vi "main.vi"() -> ()   [LabVIEW 2015]
uses:
  <vilib>/addons/_office/_exclsub.llb/font.ctl
  Keithley 2000/Public/Configure/Configure AC Volts.vi
  <vilib>/Utility/NIReport.llb/NI_report.lvclass
  Agilent 3352X Series/Agilent 3352X Series.lvlib
  Keithley 2000/Keithley 2000.lvlib
  <vilib>/addons/_office/NI_ReportGenerationToolkit.lvlib
  <vilib>/Utility/NIReport.llb/Excel/NI_Excel.lvclass
panel:
  in  "连接":bool
  out "connecting":bool
  in  "原始记录":path=path "F:/电荷放大器/2692-原始记录.xls"
  in  "2010":refnum<visa-resource-name>="GPIB0::11::INSTR"
  in  "2000":refnum<visa-resource-name>="GPIB0::16::INSTR"
  in  "channel":i32=1 min=1 max=4 step=1
  in  "COM":i32=5
  in  "退出":bool
  in  "电平":enum16{"200mV~2V", "500mV~5V"}(ring)
  in  "33521A":refnum<visa-resource-name>="USB0::0x0957::0x1607::MY50003642::INSTR"
  in  "幅频特性":bool
  in  "增益档误差":bool
  in  "归一化误差":bool
  in  "线性误差":bool
  # "电 荷 放 大 器 自 动 化"
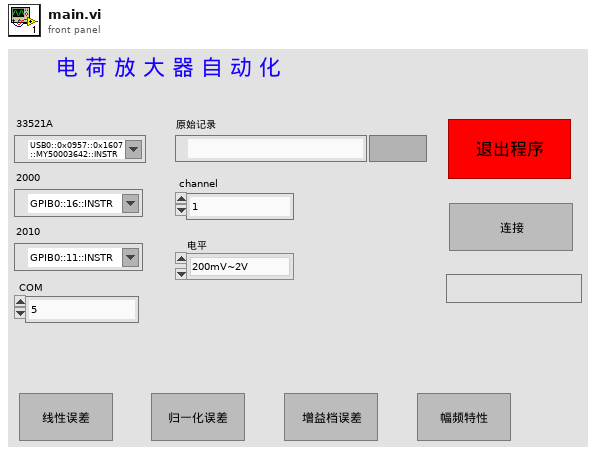
[diagram p1: front panel]
types:
  T1 = enum16{"maximized", "minimized", "normal", "no change"}
  T2 = enum16{"Standard Report", "HTML", "Word", "Excel"}
  T3 = cluster{"input float.":bool, "type":u16, "transd. mode":string, "transd. sens.":dbl, "unit":u16, "applied corr.":dbl, "position":string, "cable length":dbl, "supply":u16, "polarization":u16}
  T4 = typedef "NI_ReportGenerationToolkit.lvlib/font.ctl" = cluster{"font name":string, "font size":dbl, "bold":u16, "italic":u16, "underline":u16, "strike through":u16, "font color":u32}
  T5 = cluster{"high-pass (index)":u16, "low-pass (index)":u16, "outp. sens. (index)":u16, "output float.":bool}
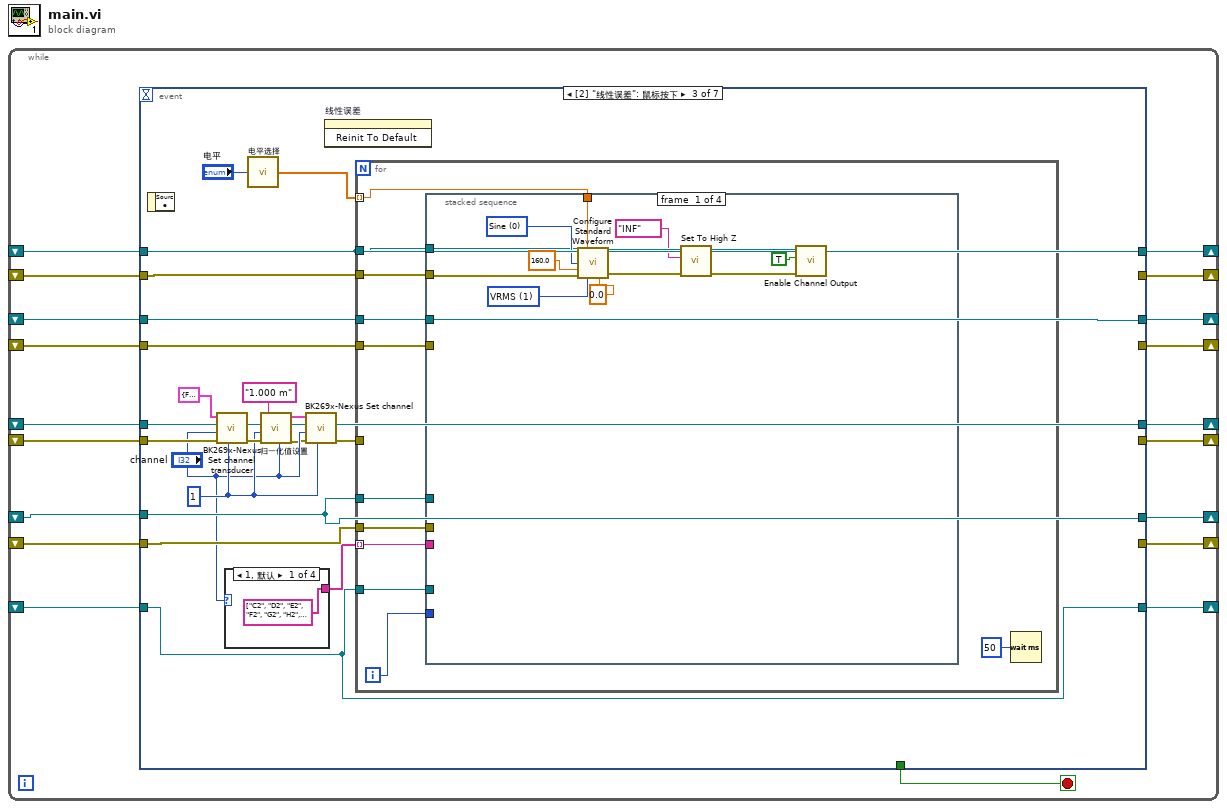
[diagram p0: block diagram]
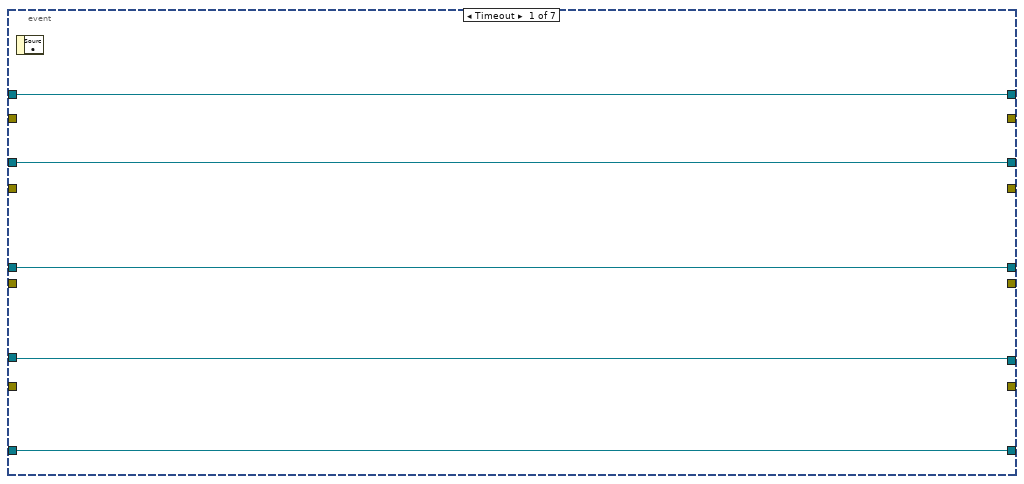
[diagram p2: hidden frame]
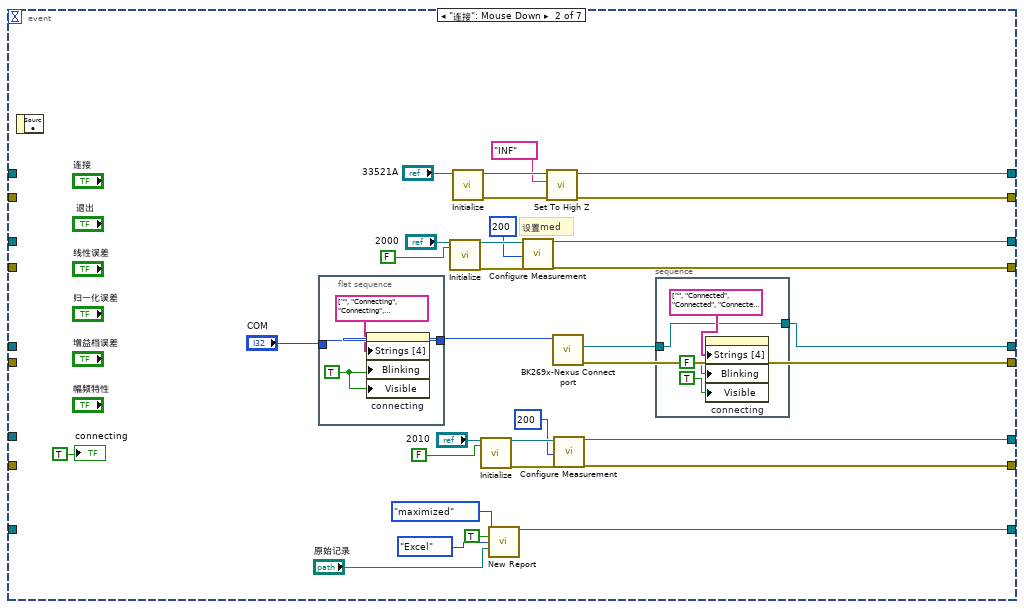
[diagram p3: hidden frame]
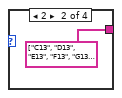
[diagram p4: hidden frame]
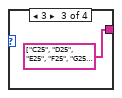
[diagram p5: hidden frame]
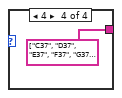
[diagram p6: hidden frame]
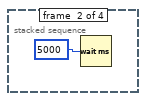
[diagram p7: hidden frame]
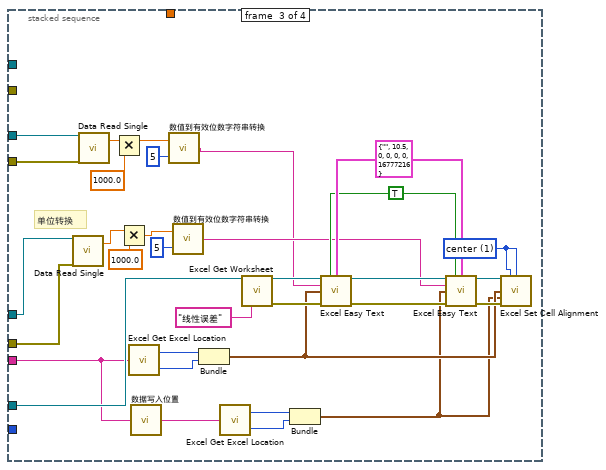
[diagram p8: hidden frame]
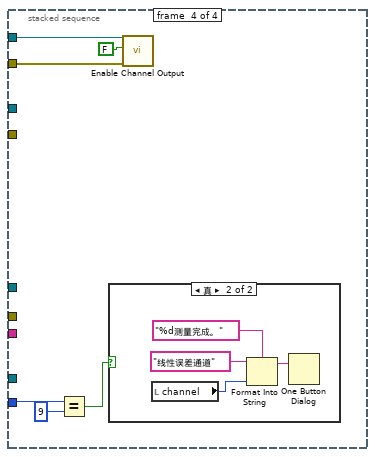
[diagram p9: hidden frame]
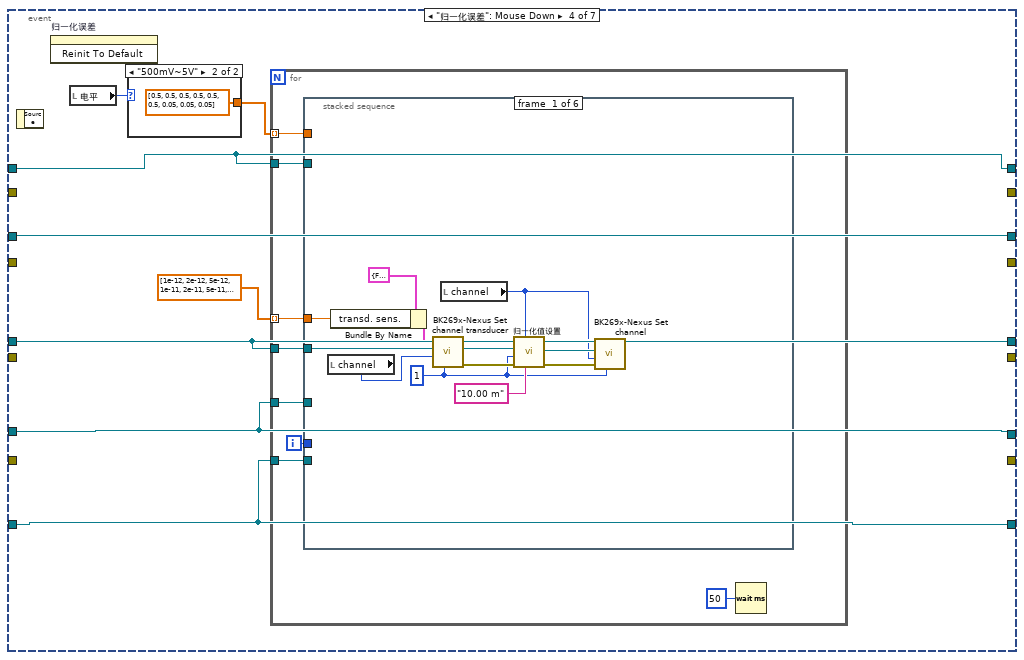
[diagram p11: hidden frame]
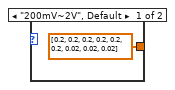
[diagram p12: hidden frame]
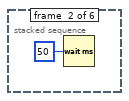
[diagram p13: hidden frame]
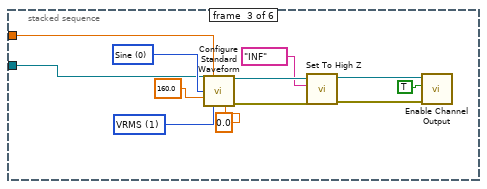
[diagram p14: hidden frame]
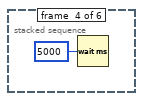
[diagram p15: hidden frame]
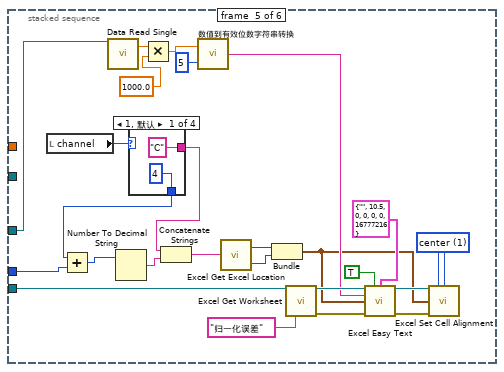
[diagram p16: hidden frame]
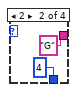
[diagram p17: hidden frame]
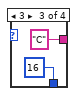
[diagram p18: hidden frame]
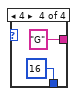
[diagram p19: hidden frame]
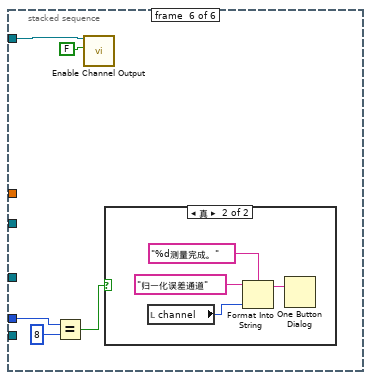
[diagram p20: hidden frame]
diagram:
  n1 = while {
    shift-right: [w18] -> _
    shift-left: _ -> [w3]
    shift-right: [w17] -> _
    shift-left: _ -> [w16]
    shift-right: [w15] -> _
    shift-left: _ -> [w14]
    shift-right: [w13] -> _
    shift-left: _ -> [w12]
    shift-right: [w11] -> _
    shift-left: _ -> [w7]
    shift-right: [w10] -> _
    shift-left: _ -> [w6]
    shift-right: [w8] -> _
    shift-left: _ -> [w1]
    shift-right: [w9] -> _
    shift-left: _ -> [w2]
    shift-right: [w5] -> _
    shift-left: _ -> [w4]
    stop <- w19 stop-if-true
    n2 = event shown="[2] \"线性误差\": 鼠标按下" {
      selector: _ -> [_ _ _ _ _ _ _]
      dyn-events: _ -> [_ _ _ _ _ _ _]
      timeout: _ -> [_ _ _ _ _ _ _]
      tunnel: [_ _ _ _ _ _ TRUE] -> w19
      tunnel: [w24 w51 w76 w160 w253 w362 w444] -> w18
      tunnel: [_ w50 _ _ _ _ _] -> w17
      tunnel: w3 -> [w24 _ w76 w160 w253 w362 w444]
      tunnel: w16 -> [_ _ w85 _ _ _ _]
      tunnel: [w20 w26 w74 w165 w254 w351 _] -> w15
      tunnel: w14 -> [w20 _ w82 w165 w254 w353 w447]
      tunnel: [_ w49 _ _ _ _ _] -> w13
      tunnel: w12 -> [_ _ w81 _ _ w352 w448]
      tunnel: [w23 w44 w75 w158 w252 w361 _] -> w11
      tunnel: [_ w43 _ _ _ _ _] -> w10
      tunnel: [w22 w38 w73 w159 w245 w355 _] -> w9
      tunnel: [_ w37 _ _ _ _ _] -> w8
      tunnel: w7 -> [w23 _ w75 w158 w252 w361 w452]
      tunnel: w6 -> [_ _ w84 _ _ _ w451]
      tunnel: [w21 w33 w72 w163 w251 w360 _] -> w5
      tunnel: w4 -> [w21 _ w72 w163 w251 w360 _]
      tunnel: w2 -> [w22 _ w73 w159 w245 w355 w450]
      tunnel: w1 -> [_ _ w79 _ _ _ w449]
      event Timeout {
        n3 = event-data() -> ()  [unwired: 1 in, 1 out]
      }
      event "连接": Mouse Down {
        # "设置med"
        n4 = event-data() -> ()  [unwired: 1 in, 1 out]
        n5 = flat-sequence {
          tunnel: "COM" -> [w60]
          tunnel: [w60] -> w28
          frame #0 {
            w61 = TRUE ("Blinking")
            n6 = property on="connecting" class="Bool (严格)"("Strings [4]"=string[] ["", "Connecting", "Connecting", "Connecting"] ("Array Constant"), "Blinking"=w61, "Visible"=w61) -> ()  [unwired: 2 in, 2 out]
          }
        }
        n7 = call "Initialize.vi"("VISA resource name"="2000", "ID Query? (T: Check)"=FALSE) -> ("VISA resource name out"=w47:refnum<visa-resource-name>, "error out"=w46:errorcluster)  [unwired: 16 in]
        n8 = call "Initialize.vi"("VISA resource name"="33521A") -> ("error out"=w55:errorcluster, "VISA resource name out"=w54:refnum<visa-resource-name>)  [unwired: 4 in, 5 out]
        n9 = call "Initialize.vi"("VISA resource name"="2010", "ID Query? (T: Check)"=FALSE) -> ("VISA resource name out"=w40:refnum<visa-resource-name>, "error out"=w41:errorcluster)  [unwired: 16 in]
        n10 = call <vilib>:"New Report.vi"("window state (normal)"=T1."maximized", "display alerts? (F)"=TRUE, "report type"=T2."Excel", "template (empty)"="原始记录") -> ("report out"=w33:refnum<class "NI_report.lvclass">)  [unwired: 10 in, 1 out]
        n11 = call-poly "Configure Measurement.vi"("VISA resource name"=w47, "Bandwidth (300 Hz)"=200, "error in (no error)"=w46) -> ("VISA resource name out"=w44:refnum<visa-resource-name>, "error out"=w43:errorcluster)  [unwired: 15 in]
        n12 = call "Set To High Z.vi"("error in (no error)"=w55, "Impedance"="INF", "VISA resource name"=w54) -> ("error out"=w50:errorcluster, "VISA resource name out"=w51:refnum<visa-resource-name>)  [unwired: 7 in]
        n13 = call <instrlib>:"BK269x-Nexus Connect port.vi"("port number"=w28) -> ("error out"=w49:errorcluster, "BKNexusD.IPort out"=w27:refnum<k7>)  [unwired: 8 in, 1 out]
        n14 = call-poly "Configure Measurement.vi"("VISA resource name"=w40, "Bandwidth (300 Hz)"=200, "error in (no error)"=w41) -> ("VISA resource name out"=w38:refnum<visa-resource-name>, "error out"=w37:errorcluster)  [unwired: 15 in]
        n15 = stacked-sequence {
          tunnel: w27 -> [w56]
          tunnel: [w56] -> w26
          frame #0 {
            n16 = property on="connecting" class="Bool (严格)"("Strings [4]"=string[] ["", "Connected", "Connected", "Connected\n"] ("Array Constant"), "Blinking"=FALSE, "Visible"=TRUE ("Blinking")) -> ()  [unwired: 2 in, 2 out]
          }
        }
        "connecting" <- TRUE ("connecting")
      }
      event "线性误差": Mouse Down {
        w68 = 1 ("amplifier")
        n17 = event-data() -> ()  [unwired: 1 in, 1 out]
        n18 = call <instrlib>:"BK269x-Nexus Set channel transducer.vi"("amplifier"=w68, "error in"=w81, "channel"="channel", "BKNexusD.IPort"=w82, "transducer information"=T3 {"input float."=FALSE, "type"=0, "transd. mode"="User", "transd. sens."=1e-12, "unit"=0, "applied corr."=1.0, "position"="", "cable length"=0.0, "supply"=0, "polarization"=65535} ("transducer settings")) -> ("error out"=w69:errorcluster, "BKNexusD.IPort"=w70:refnum<k7>)  [unwired: 4 in, 1 out]
        n19 = case shown="1, 默认" "channel" {
          tunnel: [string[] ["C2", "D2", "E2", "F2", "G2", "H2", "I2", "J2", "K2", "L2"] ("数组") string[] ["C13", "D13", "E13", "F13", "G13", "H13", "I13", "J13", "K13", "L13"] string[] ["C25", "D25", "E25", "F25", "G25", "H25", "I25", "J25", "K25", "L25"] string[] ["C37", "D37", "E37", "F37", "G37", "H37", "I37", "J37", "K37", "L37"]] -> w78
          frame 1, Default {
          }
          frame 2 {
          }
          frame 3 {
          }
          frame 4 {
          }
        }
        n20 = call "电平选择.vi"("电平输入"="电平") -> ("电平输出"=w77:dbl[])
        n21 = call "归一化值设置.vi"("归一化"="1.000 m", "channel"="channel", "错误输入（无错误）"=w69, "amplifier"=w68, "BKNexusD.IPort输入"=w70) -> ("错误输出"=w64:errorcluster, "BKNexusD.IPort输出"=w65:refnum<k7>, "channel settings"=w63:T5)  [unwired: 4 in]
        n22 = call <instrlib>:"BK269x-Nexus Set channel.vi"("amplifier"=w68, "error in"=w64, "channel"="channel", "BKNexusD.IPort"=w65, "channel settings"=w63) -> ("error out"=w80:errorcluster, "BKNexusD.IPort"=w74:refnum<k7>)  [unwired: 4 in, 1 out]
        n23 = invoke on="线性误差" class="Bool (严格)" method="Reinit To Default"() -> ()  [unwired: 3 in, 3 out]
        n24 = for {
          tunnel: w77 -> [w100] mode=indexing
          tunnel: w76 -> [w99]
          tunnel: w85 -> [w98]
          tunnel: w75 -> [w97]
          tunnel: w84 -> [w96]
          tunnel: w72 -> [w95]
          tunnel: w80 -> [_]
          tunnel: w78 -> [w94] mode=indexing
          tunnel: w73 -> [w93]
          tunnel: w79 -> [w92]
          i -> [w90]
          n25 = stacked-sequence {
            tunnel: w100 -> [w108 _ _ _]
            tunnel: w99 -> [w107 _ _ w152]
            tunnel: w98 -> [w106 _ _ w151]
            tunnel: w97 -> [_ _ w133 _]
            tunnel: w96 -> [_ _ w132 _]
            tunnel: w95 -> [_ _ w142 _]
            tunnel: w94 -> [_ _ w134 _]
            tunnel: w93 -> [_ _ w131 _]
            tunnel: w92 -> [_ _ w130 _]
            tunnel: w90 -> [_ _ _ w150]
            frame #0 {
              w110 = u16 0 items=["Sine"=0, "Square"=1, "Ramp"=2, "Noise"=3, "DC"=4, "Triangle"=5, "Pulse"=6, "Sinc"=11, "D-Lorentz"=12, "Gaussian"=13, "Expo Fall"=14, "Expo Rise"=15, "Haversine"=16] ("Waveform Function (0: Sine)")
              w113 = 1 items=["Vpp", "VRMS", "DBM"] ("Amplitude Unit (0: Vpp)")
              n26 = call "Configure Standard Waveform.vi"("VISA resource name"=w107, "Amplitude (0.1 Vpp)"=w108, "Waveform Function (0: Sine)"=w110, "Frequency/Sample Rate/Bandwidth (1000 Hz)"=160.0 ("Frequency (1000 Hz)"), "error in (no error)"=w106, "Amplitude Unit (0: Vpp)"=w113, "DC Offset (0 V)"=0.0) -> ("VISA resource name out"=w103:refnum<visa-resource-name>, "error out"=w102:errorcluster)  [unwired: 3 in, 4 out]
              n27 = call "Set To High Z.vi"("error in (no error)"=w102, "Impedance"="INF", "VISA resource name"=w103) -> ("error out"=w105:errorcluster, "VISA resource name out"=w104:refnum<visa-resource-name>)  [unwired: 7 in]
              n28 = call "Enable Channel Output.vi"("error in (no error)"=w105, "Enable Output (T: Enable)"=TRUE, "VISA resource name"=w104) -> ()  [unwired: 2 in, 7 out]
            }
            frame #1 {
              n29 = Wait (ms)(milliseconds to wait=u32 5000 ("等待时间（毫秒）")) -> ()  [unwired: 1 out]
            }
            frame #2 {
              w115 = 1 items=["left", "center", "right"] ("horizontal alignment (left)")
              w138 = TRUE ("border? (F)")
              w139 = T4 {"font name"="", "font size"=10.5, "bold"=0, "italic"=0, "underline"=0, "strike through"=0, "font color"=16777216} ("font")
              # "单位转换"
              n30 = call "Data Read Single.vi"("VISA resource name"=w131, "error in (no error)"=w130) -> ("Measurement"=w123:dbl)  [unwired: 13 in, 4 out]
              n31 = call "Data Read Single.vi"("VISA resource name"=w133, "error in (no error)"=w132) -> ("Measurement"=w128:dbl)  [unwired: 13 in, 4 out]
              n32 = Multiply(x=w128, y=1000.0) -> (x*y=w126:dbl)
              n33 = Multiply(x=w123, y=1000.0) -> (x*y=w122:dbl)
              n34 = call <vilib>:"Excel Get Excel Location.vi"("cell's name"=w134) -> ("row"=w143:i32, "column"=w144:i32)
              n35 = call "数据写入位置.vi"("标准值位置"=w134) -> ("显示值位置"=w135:string)
              n36 = call "数值到有效位数字符串转换.vi"("有效数字"=i16 5, "数值"=w126) -> ("字符串"=w120:string)
              n37 = call "数值到有效位数字符串转换.vi"("有效数字"=i16 5, "数值"=w122) -> ("字符串"=w121:string)
              n38 = Bundle("row"=w143, "column"=w144) -> (w117:cluster{"row":i32, "column":i32})  [unwired: 1 in]
              n39 = call <vilib>:"Excel Get Excel Location.vi"("cell's name"=w135) -> ("row"=w136:i32, "column"=w137:i32)
              n40 = call <vilib>:"Excel Get Worksheet.vi"("report in"=w142, "name (\"\")"="线性误差" ("name (\"\")")) -> ("report out"=w146:refnum<class "NI_report.lvclass">, "error out"=w145:errorcluster)  [unwired: 12 in]
              n41 = Bundle("row"=w136, "column"=w137) -> (w116:cluster{"row":i32, "column":i32})  [unwired: 1 in]
              n42 = call <vilib>:"Excel Easy Text.vi"("report in"=w146, "border? (F)"=w138, "font"=w139, "text"=w120, "start (-1, -1)"=w117, "error in (no error)"=w145) -> ("report out"=w140:refnum<class "NI_report.lvclass">, "error out"=w141:errorcluster)  [unwired: 5 in, 3 out]
              n43 = call <vilib>:"Excel Easy Text.vi"("report in"=w140, "border? (F)"=w138, "font"=w139, "text"=w121, "start (-1, -1)"=w116, "error in (no error)"=w141) -> ("report out"=w119:refnum<class "NI_report.lvclass">, "error out"=w118:errorcluster)  [unwired: 5 in, 3 out]
              n44 = call <vilib>:"Excel Set Cell Alignment.vi"("report in"=w119, "vertical alignment (top)"=w115, "horizontal alignment (left)"=w115, "start (-1, -1)"=w117, "end (-1, -1)"=w116, "error in (no error)"=w118) -> ()  [unwired: 8 in, 2 out]
            }
            frame #3 {
              n45 = Equal?(x=w150, y=9) -> (x = y?=w148:bool)
              n46 = case shown="真" w148 {
                frame False {
                }
                frame True {
                  n47 = local read "channel"() -> (w156:i32)
                  n48 = Format Into String(format string="%d测量完成。" ("格式字符串"), initial string="线性误差通道" ("name (\"\")"), w156) -> (resulting string=w154:string)  [unwired: 1 in, 1 out]
                  n49 = One Button Dialog(message=w154) -> ()  [unwired: 1 in, 1 out]
                }
              }
              n50 = call "Enable Channel Output.vi"("error in (no error)"=w151, "Enable Output (T: Enable)"=FALSE, "VISA resource name"=w152) -> ()  [unwired: 2 in, 7 out]
            }
          }
          n51 = Wait (ms)(milliseconds to wait=u32 50 ("等待时间（毫秒）")) -> ()  [unwired: 1 out]
        }
      }
      event "归一化误差": Mouse Down {
        n52 = event-data() -> ()  [unwired: 1 in, 1 out]
        n53 = invoke on="归一化误差" class="Bool (严格)" method="Reinit To Default"() -> ()  [unwired: 3 in, 3 out]
        n54 = local read "电平"() -> (w162:enum16{"200mV~2V", "500mV~5V"})
        n55 = case shown="\"500mV~5V\"" w162 {
          tunnel: [dbl[] [0.2, 0.2, 0.2, 0.2, 0.2, 0.2, 0.02, 0.02, 0.02] dbl[] [0.5, 0.5, 0.5, 0.5, 0.5, 0.5, 0.05, 0.05, 0.05]] -> w161
          frame "200mV~2V", Default {
          }
          frame "500mV~5V" {
          }
        }
        n56 = for {
          tunnel: w165 -> [w175]
          tunnel: dbl[] [1e-12, 2e-12, 5e-12, 1e-11, 2e-11, 5e-11, 1e-13, 2e-13, 5e-13] -> [w174] mode=indexing
          tunnel: w163 -> [w172]
          tunnel: w161 -> [w170] mode=indexing
          tunnel: w160 -> [w169]
          tunnel: w159 -> [w168]
          i -> [w171]
          n57 = stacked-sequence {
            tunnel: w175 -> [w187 _ _ _ _ _]
            tunnel: w174 -> [w186 _ _ _ _ _]
            tunnel: w169 -> [_ _ w191 _ _ w239]
            tunnel: w172 -> [_ _ _ _ w220 _]
            tunnel: w171 -> [_ _ _ _ w214 w236]
            tunnel: w170 -> [_ _ w190 _ _ _]
            tunnel: w168 -> [_ _ _ _ w207 _]
            frame #0 {
              w176 = 1 ("amplifier")
              n58 = local read "channel"() -> (w184:i32)
              n59 = Bundle By Name(cluster=T3 {"input float."=FALSE, "type"=0, "transd. mode"="User", "transd. sens."=1e-12, "unit"=0, "applied corr."=1.0, "position"="", "cable length"=0.0, "supply"=0, "polarization"=65535} ("transducer settings"), "transd. sens."=w186) -> (w185:T3)
              n60 = call <instrlib>:"BK269x-Nexus Set channel transducer.vi"("amplifier"=w176, "channel"=w184, "BKNexusD.IPort"=w187, "transducer information"=w185) -> ("error out"=w182:errorcluster, "BKNexusD.IPort"=w183:refnum<k7>)  [unwired: 5 in, 1 out]
              n61 = local read "channel"() -> (w177:i32)
              n62 = call "归一化值设置.vi"("归一化"="10.00 m", "channel"=w177, "错误输入（无错误）"=w182, "amplifier"=w176, "BKNexusD.IPort输入"=w183) -> ("错误输出"=w180:errorcluster, "BKNexusD.IPort输出"=w178:refnum<k7>, "channel settings"=w179:T5)  [unwired: 4 in]
              n63 = call <instrlib>:"BK269x-Nexus Set channel.vi"("amplifier"=w176, "error in"=w180, "channel"=w177, "BKNexusD.IPort"=w178, "channel settings"=w179) -> ()  [unwired: 4 in, 3 out]
            }
            frame #1 {
              n64 = Wait (ms)(milliseconds to wait=u32 50 ("等待时间（毫秒）")) -> ()  [unwired: 1 out]
            }
            frame #2 {
              w198 = u16 0 items=["Sine"=0, "Square"=1, "Ramp"=2, "Noise"=3, "DC"=4, "Triangle"=5, "Pulse"=6, "Sinc"=11, "D-Lorentz"=12, "Gaussian"=13, "Expo Fall"=14, "Expo Rise"=15, "Haversine"=16] ("Waveform Function (0: Sine)")
              w201 = 1 items=["Vpp", "VRMS", "DBM"] ("Amplitude Unit (0: Vpp)")
              n65 = call "Configure Standard Waveform.vi"("VISA resource name"=w191, "Amplitude (0.1 Vpp)"=w190, "Waveform Function (0: Sine)"=w198, "Frequency/Sample Rate/Bandwidth (1000 Hz)"=160.0 ("Frequency (1000 Hz)"), "Amplitude Unit (0: Vpp)"=w201, "DC Offset (0 V)"=0.0) -> ("VISA resource name out"=w194:refnum<visa-resource-name>, "error out"=w193:errorcluster)  [unwired: 4 in, 4 out]
              n66 = call "Set To High Z.vi"("error in (no error)"=w193, "Impedance"="INF", "VISA resource name"=w194) -> ("error out"=w196:errorcluster, "VISA resource name out"=w195:refnum<visa-resource-name>)  [unwired: 7 in]
              n67 = call "Enable Channel Output.vi"("error in (no error)"=w196, "Enable Output (T: Enable)"=TRUE, "VISA resource name"=w195) -> ()  [unwired: 2 in, 7 out]
            }
            frame #3 {
              n68 = Wait (ms)(milliseconds to wait=u32 5000 ("等待时间（毫秒）")) -> ()  [unwired: 1 out]
            }
            frame #4 {
              w204 = 1 items=["top", "center", "bottom"] ("vertical alignment (top)")
              n69 = local read "channel"() -> (w210:i32)
              n70 = call "Data Read Single.vi"("VISA resource name"=w207) -> ("Measurement"=w226:dbl)  [unwired: 14 in, 4 out]
              n71 = case shown="1, 默认" w210 {
                tunnel: ["C" ("name (\"\")") "G" ("name (\"\")") "C" ("name (\"\")") "G" ("name (\"\")")] -> w208
                tunnel: [4 ("y") 4 ("y") 16 ("y") 16 ("y")] -> w209
                frame 1, Default {
                }
                frame 2 {
                }
                frame 3 {
                }
                frame 4 {
                }
              }
              n72 = Add(x=w209, y=w214) -> (x+y=w213:i32)
              n73 = Number To Decimal String(number=w213) -> (decimal integer string=w212:string)  [unwired: 1 in]
              n74 = Multiply(x=w226, y=1000.0) -> (x*y=w225:dbl)
              n75 = Concatenate Strings(w208, w212) -> (w211:string)
              n76 = call "数值到有效位数字符串转换.vi"("有效数字"=i16 5, "数值"=w225) -> ("字符串"=w219:string)
              n77 = call <vilib>:"Excel Get Excel Location.vi"("cell's name"=w211) -> ("row"=w217:i32, "column"=w218:i32)
              n78 = Bundle("row"=w217, "column"=w218) -> (w203:cluster{"row":i32, "column":i32})  [unwired: 1 in]
              n79 = call <vilib>:"Excel Get Worksheet.vi"("report in"=w220, "name (\"\")"="归一化误差" ("name (\"\")")) -> ("report out"=w222:refnum<class "NI_report.lvclass">, "error out"=w221:errorcluster)  [unwired: 12 in]
              n80 = call <vilib>:"Excel Easy Text.vi"("report in"=w222, "border? (F)"=TRUE, "font"=T4 {"font name"="", "font size"=10.5, "bold"=0, "italic"=0, "underline"=0, "strike through"=0, "font color"=16777216}, "text"=w219, "start (-1, -1)"=w203, "error in (no error)"=w221) -> ("report out"=w206:refnum<class "NI_report.lvclass">, "error out"=w205:errorcluster)  [unwired: 5 in, 3 out]
              n81 = call <vilib>:"Excel Set Cell Alignment.vi"("report in"=w206, "vertical alignment (top)"=w204, "horizontal alignment (left)"=w204, "start (-1, -1)"=w203, "error in (no error)"=w205) -> ()  [unwired: 9 in, 2 out]
            }
            frame #5 {
              n82 = Equal?(x=w236, y=8) -> (x = y?=w237:bool)
              n83 = call "Enable Channel Output.vi"("Enable Output (T: Enable)"=FALSE, "VISA resource name"=w239) -> ()  [unwired: 3 in, 7 out]
              n84 = case shown="真" w237 {
                frame False {
                }
                frame True {
                  n85 = local read "channel"() -> (w243:i32)
                  n86 = Format Into String(format string="%d测量完成。" ("格式字符串"), initial string="归一化误差通道" ("name (\"\")"), w243) -> (resulting string=w241:string)  [unwired: 1 in, 1 out]
                  n87 = One Button Dialog(message=w241) -> ()  [unwired: 1 in, 1 out]
                }
              }
            }
          }
          n88 = Wait (ms)(milliseconds to wait=u32 50 ("等待时间（毫秒）")) -> ()  [unwired: 1 out]
        }
      }
      event "增益档误差": Mouse Down {
        n89 = event-data() -> ()  [unwired: 1 in, 1 out]
        n90 = local read "channel"() -> (w247:i32)
        n91 = local read "电平"() -> (w249:enum16{"200mV~2V", "500mV~5V"})
        n92 = invoke on="增益档误差" class="Bool (严格)" method="Reinit To Default"() -> ()  [unwired: 3 in, 3 out]
        n93 = case shown="\"500mV~5V\"" w249 {
          tunnel: [dbl[] [2.0, 0.63, 2.0, 0.63, 0.2, 0.63, 0.2, 0.63, 0.2] dbl[] [5.0, 1.58, 5.0, 1.58, 0.5, 1.58, 0.5, 1.58, 0.5]] -> w248
          frame "200mV~2V", Default {
          }
          frame "500mV~5V" {
          }
        }
        n94 = case shown="1, 默认" w247 {
          tunnel: [string[] ["C4", "D4", "E4", "F4", "G4", "C10", "D10", "E10", "F10"] string[] ["C18", "D18", "E18", "F18", "G18", "C24", "D24", "E24", "F24"] string[] ["C31", "D31", "E31", "F31", "G31", "C37", "D37", "E37", "F37"] string[] ["C44", "D44", "E44", "F44", "G44", "C50", "D50", "E50", "F50"]] -> w246
          frame 1, Default {
          }
          frame 2 {
          }
          frame 3 {
          }
          frame 4 {
          }
        }
        n95 = for {
          tunnel: w254 -> [w270]
          tunnel: dbl[] [1e-13, 1e-13, 1e-12, 1e-12, 1e-12, 1e-11, 1e-11, 1e-10, 1e-10] -> [w269] mode=indexing
          tunnel: w253 -> [w267]
          tunnel: w252 -> [w266]
          tunnel: w251 -> [w265]
          tunnel: w248 -> [w263] mode=indexing
          tunnel: w246 -> [w262] mode=indexing
          tunnel: w245 -> [w261]
          i -> [w264]
          n96 = stacked-sequence {
            tunnel: w270 -> [w286 _ _ _ _ _]
            tunnel: w269 -> [w285 _ _ _ _ _]
            tunnel: w267 -> [_ _ w290 _ _ w336]
            tunnel: w266 -> [_ _ _ _ w328 _]
            tunnel: w265 -> [_ _ _ _ w324 _]
            tunnel: w264 -> [w278 _ _ _ _ w333]
            tunnel: w263 -> [_ _ w289 _ _ _]
            tunnel: w262 -> [_ _ _ _ w318 _]
            tunnel: w261 -> [_ _ _ _ w312 _]
            frame #0 {
              w280 = 1 ("amplifier")
              n97 = local read "channel"() -> (w283:i32)
              n98 = Bundle By Name(cluster=T3 {"input float."=FALSE, "type"=0, "transd. mode"="User", "transd. sens."=1e-12, "unit"=0, "applied corr."=1.0, "position"="", "cable length"=0.0, "supply"=0, "polarization"=65535} ("transducer settings"), "transd. sens."=w285) -> (w284:T3)
              n99 = Index Array(array=string[] ["100.0 u", "316.2 u", "1.000 m", "3.162 m", "10.00 m", "31.62 m", "100.0 m", "316.2 m", "1.000  "], index=w278) -> (element=w271:string)
              n100 = call <instrlib>:"BK269x-Nexus Set channel transducer.vi"("amplifier"=w280, "channel"=w283, "BKNexusD.IPort"=w286, "transducer information"=w284) -> ("error out"=w281:errorcluster, "BKNexusD.IPort"=w282:refnum<k7>)  [unwired: 5 in, 1 out]
              n101 = local read "channel"() -> (w272:i32)
              n102 = call "归一化值设置.vi"("归一化"=w271, "channel"=w272, "错误输入（无错误）"=w281, "amplifier"=w280, "BKNexusD.IPort输入"=w282) -> ("错误输出"=w273:errorcluster, "BKNexusD.IPort输出"=w274:refnum<k7>, "channel settings"=w275:T5)  [unwired: 4 in]
              n103 = local read "channel"() -> (w276:i32)
              n104 = call <instrlib>:"BK269x-Nexus Set channel.vi"("amplifier"=1, "error in"=w273, "channel"=w276, "BKNexusD.IPort"=w274, "channel settings"=w275) -> ()  [unwired: 4 in, 3 out]
            }
            frame #1 {
              n105 = Wait (ms)(milliseconds to wait=u32 50 ("等待时间（毫秒）")) -> ()  [unwired: 1 out]
            }
            frame #2 {
              w297 = u16 0 items=["Sine"=0, "Square"=1, "Ramp"=2, "Noise"=3, "DC"=4, "Triangle"=5, "Pulse"=6, "Sinc"=11, "D-Lorentz"=12, "Gaussian"=13, "Expo Fall"=14, "Expo Rise"=15, "Haversine"=16] ("Waveform Function (0: Sine)")
              w300 = 1 items=["Vpp", "VRMS", "DBM"] ("Amplitude Unit (0: Vpp)")
              n106 = call "Configure Standard Waveform.vi"("VISA resource name"=w290, "Amplitude (0.1 Vpp)"=w289, "Waveform Function (0: Sine)"=w297, "Frequency/Sample Rate/Bandwidth (1000 Hz)"=160.0 ("Frequency (1000 Hz)"), "Amplitude Unit (0: Vpp)"=w300, "DC Offset (0 V)"=0.0) -> ("VISA resource name out"=w293:refnum<visa-resource-name>, "error out"=w292:errorcluster)  [unwired: 4 in, 4 out]
              n107 = call "Set To High Z.vi"("error in (no error)"=w292, "Impedance"="INF", "VISA resource name"=w293) -> ("error out"=w295:errorcluster, "VISA resource name out"=w294:refnum<visa-resource-name>)  [unwired: 7 in]
              n108 = call "Enable Channel Output.vi"("error in (no error)"=w295, "Enable Output (T: Enable)"=TRUE, "VISA resource name"=w294) -> ()  [unwired: 2 in, 7 out]
            }
            frame #3 {
              n109 = Wait (ms)(milliseconds to wait=u32 5000 ("等待时间（毫秒）")) -> ()  [unwired: 1 out]
            }
            frame #4 {
              w302 = 1 items=["top", "center", "bottom"] ("vertical alignment (top)")
              w311 = T4 {"font name"="", "font size"=10.5, "bold"=0, "italic"=0, "underline"=0, "strike through"=0, "font color"=16777216} ("font")
              w310 = TRUE ("border? (F)")
              n110 = call "Data Read Single.vi"("VISA resource name"=w328) -> ("Measurement"=w331:dbl)  [unwired: 14 in, 4 out]
              n111 = call <vilib>:"Excel Get Excel Location.vi"("cell's name"=w318) -> ("row"=w322:i32, "column"=w323:i32)
              n112 = call "Data Read Single.vi"("VISA resource name"=w312) -> ("Measurement"=w314:dbl)  [unwired: 14 in, 4 out]
              n113 = Multiply(x=w331, y=1000.0) -> (x*y=w330:dbl)
              n114 = Multiply(x=w314, y=1000.0) -> (x*y=w315:dbl)
              n115 = call <vilib>:"Excel Get Worksheet.vi"("report in"=w324, "name (\"\")"="增益档误差" ("name (\"\")")) -> ("report out"=w326:refnum<class "NI_report.lvclass">, "error out"=w325:errorcluster)  [unwired: 12 in]
              n116 = Bundle("row"=w322, "column"=w323) -> (w304:cluster{"row":i32, "column":i32})  [unwired: 1 in]
              n117 = call "数值到有效位数字符串转换.vi"("有效数字"=i16 5, "数值"=w330) -> ("字符串"=w307:string)
              n118 = call "数值到有效位数字符串转换.vi"("有效数字"=i16 5, "数值"=w315) -> ("字符串"=w308:string)
              n119 = call "数据写入位置.vi"("标准值位置"=w318) -> ("显示值位置"=w319:string)
              n120 = call <vilib>:"Excel Easy Text.vi"("report in"=w326, "border? (F)"=w310, "font"=w311, "text"=w307, "start (-1, -1)"=w304, "error in (no error)"=w325) -> ("report out"=w317:refnum<class "NI_report.lvclass">, "error out"=w309:errorcluster)  [unwired: 5 in, 3 out]
              n121 = call <vilib>:"Excel Get Excel Location.vi"("cell's name"=w319) -> ("row"=w320:i32, "column"=w321:i32)
              n122 = Bundle("row"=w320, "column"=w321) -> (w303:cluster{"row":i32, "column":i32})  [unwired: 1 in]
              n123 = call <vilib>:"Excel Easy Text.vi"("report in"=w317, "border? (F)"=w310, "font"=w311, "text"=w308, "start (-1, -1)"=w303, "error in (no error)"=w309) -> ("report out"=w306:refnum<class "NI_report.lvclass">, "error out"=w305:errorcluster)  [unwired: 5 in, 3 out]
              n124 = call <vilib>:"Excel Set Cell Alignment.vi"("report in"=w306, "vertical alignment (top)"=w302, "horizontal alignment (left)"=w302, "start (-1, -1)"=w304, "end (-1, -1)"=w303, "error in (no error)"=w305) -> ()  [unwired: 8 in, 2 out]
            }
            frame #5 {
              n125 = Equal?(x=w333, y=8) -> (x = y?=w334:bool)
              n126 = call "Enable Channel Output.vi"("Enable Output (T: Enable)"=FALSE, "VISA resource name"=w336) -> ()  [unwired: 3 in, 7 out]
              n127 = case shown="真" w334 {
                frame False {
                }
                frame True {
                  n128 = local read "channel"() -> (w340:i32)
                  n129 = Format Into String(format string="%d测量完成。" ("格式字符串"), initial string="增益档误差" ("name (\"\")"), w340) -> (resulting string=w338:string)  [unwired: 1 in, 1 out]
                  n130 = One Button Dialog(message=w338) -> ()  [unwired: 1 in, 1 out]
                }
              }
            }
          }
          n131 = Wait (ms)(milliseconds to wait=u32 50 ("等待时间（毫秒）")) -> ()  [unwired: 1 out]
        }
      }
      event "幅频特性": Mouse Down {
        w347 = 1 ("amplifier")
        n132 = event-data() -> ()  [unwired: 1 in, 1 out]
        n133 = local read "channel"() -> (w357:i32)
        n134 = local read "channel"() -> (w346:i32)
        n135 = invoke on="幅频特性" class="Bool (严格)" method="Reinit To Default"() -> ()  [unwired: 3 in, 3 out]
        n136 = case shown="1, 默认" w357 {
          tunnel: [string[] ["C4", "D4", "E4", "F4", "G4", "H4", "I4", "J4", "K4", "L4"] string[] ["C11", "D11", "E11", "F11", "G11", "H11", "I11", "J11", "K11", "L11"] string[] ["C18", "D18", "E18", "F18", "G18", "H18", "I18", "J18", "K18", "L18"] string[] ["C25", "D25", "E25", "F25", "G25", "H25", "I25", "J25", "K25", "L25"]] -> w356
          frame 1, Default {
          }
          frame 2 {
          }
          frame 3 {
          }
          frame 4 {
          }
        }
        n137 = call <instrlib>:"BK269x-Nexus Set channel transducer.vi"("amplifier"=w347, "error in"=w352, "channel"=w346, "BKNexusD.IPort"=w353, "transducer information"=T3 {"input float."=FALSE, "type"=0, "transd. mode"="User", "transd. sens."=1e-12, "unit"=0, "applied corr."=1.0, "position"="", "cable length"=0.0, "supply"=0, "polarization"=65535} ("transducer settings")) -> ("error out"=w348:errorcluster, "BKNexusD.IPort"=w349:refnum<k7>)  [unwired: 4 in, 1 out]
        n138 = local read "电平"() -> (w359:enum16{"200mV~2V", "500mV~5V"})
        n139 = call "归一化值设置.vi"("归一化"="1.000 m", "channel"=w346, "错误输入（无错误）"=w348, "amplifier"=w347, "BKNexusD.IPort输入"=w349) -> ("错误输出"=w343:errorcluster, "BKNexusD.IPort输出"=w344:refnum<k7>, "channel settings"=w342:T5)  [unwired: 4 in]
        n140 = case shown="\"500mV~5V\"" w359 {
          tunnel: [2.0 5.0] -> w358
          frame "200mV~2V", Default {
          }
          frame "500mV~5V" {
          }
        }
        n141 = call <instrlib>:"BK269x-Nexus Set channel.vi"("amplifier"=w347, "error in"=w343, "channel"=w346, "BKNexusD.IPort"=w344, "channel settings"=w342) -> ("BKNexusD.IPort"=w351:refnum<k7>)  [unwired: 4 in, 2 out]
        n142 = for {
          tunnel: w362 -> [w376]
          tunnel: w361 -> [w375]
          tunnel: w360 -> [w374]
          tunnel: w358 -> [w373]
          tunnel: w356 -> [w372] mode=indexing
          tunnel: w355 -> [w371]
          tunnel: dbl[] [10.0, 20.0, 40.0, 80.0, 160.0, 640.0, 1000.0, 2000.0, 5000.0, 8000.0] -> [w370] mode=indexing
          i -> [w369]
          n143 = stacked-sequence {
            tunnel: w376 -> [w380 _ _ w438]
            tunnel: w375 -> [_ w391 w430 _]
            tunnel: w374 -> [_ _ w426 _]
            tunnel: w373 -> [w379 _ _ _]
            tunnel: w372 -> [_ _ w420 _]
            tunnel: w371 -> [_ w390 w414 _]
            tunnel: w370 -> [w378 _ _ _]
            tunnel: w369 -> [_ w393 _ w435]
            frame #0 {
              w386 = u16 0 items=["Sine"=0, "Square"=1, "Ramp"=2, "Noise"=3, "DC"=4, "Triangle"=5, "Pulse"=6, "Sinc"=11, "D-Lorentz"=12, "Gaussian"=13, "Expo Fall"=14, "Expo Rise"=15, "Haversine"=16] ("Waveform Function (0: Sine)")
              w389 = 1 items=["Vpp", "VRMS", "DBM"] ("Amplitude Unit (0: Vpp)")
              n144 = call "Configure Standard Waveform.vi"("VISA resource name"=w380, "Amplitude (0.1 Vpp)"=w379, "Waveform Function (0: Sine)"=w386, "Frequency/Sample Rate/Bandwidth (1000 Hz)"=w378, "Amplitude Unit (0: Vpp)"=w389, "DC Offset (0 V)"=0.0) -> ("VISA resource name out"=w383:refnum<visa-resource-name>, "error out"=w382:errorcluster)  [unwired: 4 in, 4 out]
              n145 = call "Set To High Z.vi"("error in (no error)"=w382, "Impedance"="INF", "VISA resource name"=w383) -> ("error out"=w385:errorcluster, "VISA resource name out"=w384:refnum<visa-resource-name>)  [unwired: 7 in]
              n146 = call "Enable Channel Output.vi"("error in (no error)"=w385, "Enable Output (T: Enable)"=TRUE, "VISA resource name"=w384) -> ()  [unwired: 2 in, 7 out]
            }
            frame #1 {
              n147 = case shown="2, 默认" w393 {
                tunnel: [u32 5000 ("等待时间（毫秒）") u32 10000 ("等待时间（毫秒）")] -> w392
                tunnel: w391 -> [w396 w401]
                tunnel: w390 -> [w394 w399]
                frame 2, Default {
                  n148 = call-poly "Configure Measurement.vi"("VISA resource name"=w396, "Bandwidth (300 Hz)"=200) -> ()  [unwired: 16 in, 2 out]
                  n149 = call-poly "Configure Measurement.vi"("VISA resource name"=w394, "Bandwidth (300 Hz)"=200) -> ()  [unwired: 16 in, 2 out]
                }
                frame 0, 1 {
                  # "slow"
                  n150 = call-poly "Configure Measurement.vi"("VISA resource name"=w401, "Bandwidth (300 Hz)"=20) -> ()  [unwired: 16 in, 2 out]
                  n151 = call-poly "Configure Measurement.vi"("VISA resource name"=w399, "Bandwidth (300 Hz)"=20) -> ()  [unwired: 16 in, 2 out]
                }
              }
              n152 = Wait (ms)(milliseconds to wait=w392) -> ()  [unwired: 1 out]
            }
            frame #2 {
              w404 = 1 items=["top", "center", "bottom"] ("vertical alignment (top)")
              w413 = T4 {"font name"="", "font size"=10.5, "bold"=0, "italic"=0, "underline"=0, "strike through"=0, "font color"=16777216} ("font")
              w412 = TRUE ("border? (F)")
              n153 = call "Data Read Single.vi"("VISA resource name"=w430) -> ("Measurement"=w433:dbl)  [unwired: 14 in, 4 out]
              n154 = call <vilib>:"Excel Get Excel Location.vi"("cell's name"=w420) -> ("row"=w424:i32, "column"=w425:i32)
              n155 = call "Data Read Single.vi"("VISA resource name"=w414) -> ("Measurement"=w416:dbl)  [unwired: 14 in, 4 out]
              n156 = Multiply(x=w433, y=1000.0) -> (x*y=w432:dbl)
              n157 = Multiply(x=w416, y=1000.0) -> (x*y=w417:dbl)
              n158 = call <vilib>:"Excel Get Worksheet.vi"("report in"=w426, "name (\"\")"="幅频特性" ("name (\"\")")) -> ("report out"=w428:refnum<class "NI_report.lvclass">, "error out"=w427:errorcluster)  [unwired: 12 in]
              n159 = Bundle("row"=w424, "column"=w425) -> (w406:cluster{"row":i32, "column":i32})  [unwired: 1 in]
              n160 = call "数值到有效位数字符串转换.vi"("有效数字"=i16 5, "数值"=w432) -> ("字符串"=w409:string)
              n161 = call "数值到有效位数字符串转换.vi"("有效数字"=i16 5, "数值"=w417) -> ("字符串"=w410:string)
              n162 = call "数据写入位置.vi"("标准值位置"=w420) -> ("显示值位置"=w421:string)
              n163 = call <vilib>:"Excel Easy Text.vi"("report in"=w428, "border? (F)"=w412, "font"=w413, "text"=w409, "start (-1, -1)"=w406, "error in (no error)"=w427) -> ("report out"=w419:refnum<class "NI_report.lvclass">, "error out"=w411:errorcluster)  [unwired: 5 in, 3 out]
              n164 = call <vilib>:"Excel Get Excel Location.vi"("cell's name"=w421) -> ("row"=w422:i32, "column"=w423:i32)
              n165 = Bundle("row"=w422, "column"=w423) -> (w405:cluster{"row":i32, "column":i32})  [unwired: 1 in]
              n166 = call <vilib>:"Excel Easy Text.vi"("report in"=w419, "border? (F)"=w412, "font"=w413, "text"=w410, "start (-1, -1)"=w405, "error in (no error)"=w411) -> ("report out"=w408:refnum<class "NI_report.lvclass">, "error out"=w407:errorcluster)  [unwired: 5 in, 3 out]
              n167 = call <vilib>:"Excel Set Cell Alignment.vi"("report in"=w408, "vertical alignment (top)"=w404, "horizontal alignment (left)"=w404, "start (-1, -1)"=w406, "end (-1, -1)"=w405, "error in (no error)"=w407) -> ()  [unwired: 8 in, 2 out]
            }
            frame #3 {
              n168 = call "Enable Channel Output.vi"("Enable Output (T: Enable)"=FALSE, "VISA resource name"=w438) -> ()  [unwired: 3 in, 7 out]
              n169 = Equal?(x=w435, y=9) -> (x = y?=w436:bool)
              n170 = case shown="真" w436 {
                frame False {
                }
                frame True {
                  n171 = local read "channel"() -> (w442:i32)
                  n172 = Format Into String(format string="%d测量完成。" ("格式字符串"), initial string="幅频特性" ("name (\"\")"), w442) -> (resulting string=w440:string)  [unwired: 1 in, 1 out]
                  n173 = One Button Dialog(message=w440) -> ()  [unwired: 1 in, 1 out]
                }
              }
            }
          }
          n174 = Wait (ms)(milliseconds to wait=u32 50 ("等待时间（毫秒）")) -> ()  [unwired: 1 out]
        }
      }
      event "退出": Mouse Down {
        n175 = event-data() -> ()  [unwired: 1 in, 1 out]
        n176 = invoke on="退出" class="Bool (严格)" method="Reinit To Default"() -> ()  [unwired: 3 in, 3 out]
        n177 = call "Close.vi"("VISA resource name"=w450, "error in (no error)"=w449) -> ()  [unwired: 17 in, 1 out]
        n178 = call "Close.vi"("VISA resource name"=w452, "error in (no error)"=w451) -> ()  [unwired: 17 in, 1 out]
        n179 = flat-sequence {
          tunnel: w447 -> [w457]
          tunnel: [w457] -> w446
          frame #0 {
            w459 = TRUE ("Blinking")
            n180 = property on="connecting" class="Bool (严格)"("Strings [4]"=string[] ["", "Disconnecting", "", ""] ("Array Constant"), "Blinking"=w459, "Visible"=w459) -> ()  [unwired: 2 in, 2 out]
          }
        }
        n181 = invoke on="连接" class="Bool (严格)" method="Reinit To Default"() -> ()  [unwired: 3 in, 3 out]
        n182 = call <instrlib>:"BK269x-Nexus Disconnect port.vi"("error in"=w448, "BKNexusD.IPort"=w446) -> ("error out"=w445:errorcluster)  [unwired: 9 in]
        n183 = flat-sequence {
          tunnel: w445 -> [_]
          frame #0 {
            n184 = property on="connecting" class="Bool (严格)"("Strings [4]"=string[] ["", "Disconnecting", "", ""] ("Array Constant"), "Blinking"=FALSE, "Visible"=TRUE ("Blinking")) -> ()  [unwired: 2 in, 2 out]
          }
        }
      }
    }
  }
